vi "sectors checker.vi"(8 "error in (no error)":errorcluster, 10 "sections 2":string[][](array[string]), 11 "sections 1":string[][](array[string])) -> (0 "error out":errorcluster)   [LabVIEW 2024]
doc: "This VI compares the sections of two configuration files. The section names from each file are stored in the arrays <b>sections 1</b> and <b>sections 2</b>."
uses:
  443d4004-14de-444d-9e4b-623f00349db9.vi
  <vilib>/Utility/error.llb/Error Cluster From Error Code.vi
  <vilib>/ErrorRing/Error Ring.xnode
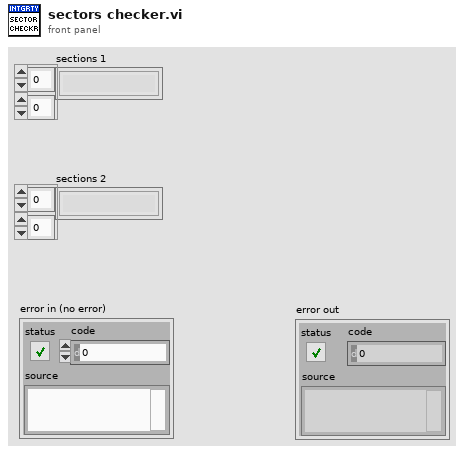
[diagram p1: front panel]
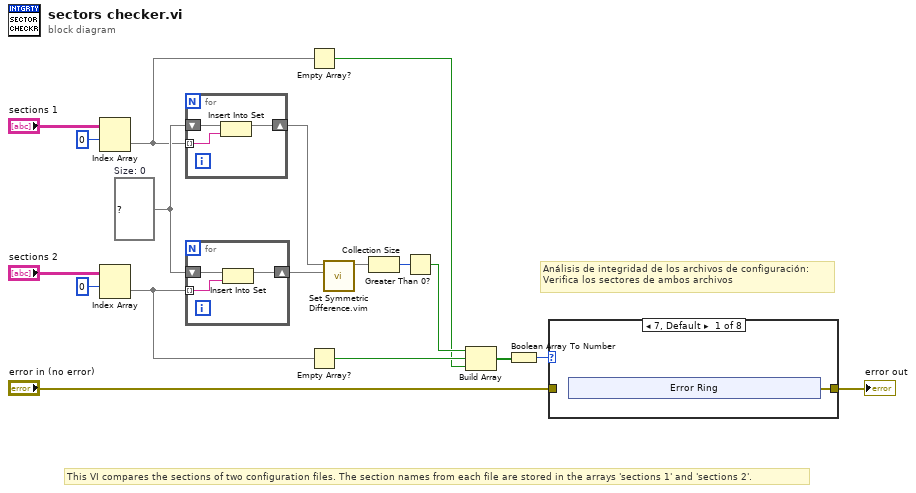
[diagram p0: block diagram]
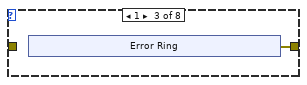
[diagram p3: hidden frame]
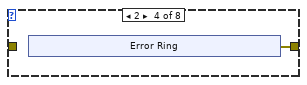
[diagram p4: hidden frame]
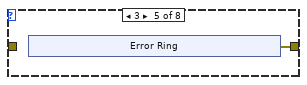
[diagram p5: hidden frame]
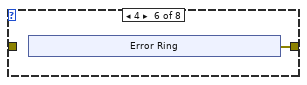
[diagram p6: hidden frame]
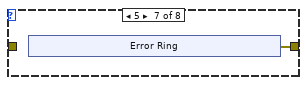
[diagram p7: hidden frame]
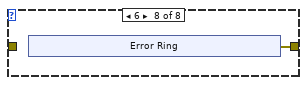
[diagram p8: hidden frame]
diagram:
  w15 = set{string} {}  # Size: 0
  # "This VI compares the sections of two configuration files. The section names from each file are stored in the arrays 'sections 1' and 'sections 2'."
  # "Análisis de integridad de los archivos de configuración:\nVerifica los sectores de ambos archivos"
  n1 = Index Array(array="sections 1", index (row)=0) -> (element=w1:string[])  [unwired: 1 in]
  n2 = Index Array(array="sections 2", index (row)=0) -> (element=w4:string[])  [unwired: 1 in]
  n3 = for {
    shift-right: [w20] -> w14
    shift-left: w15 -> [w21]
    tunnel: w1 -> [w19] mode=indexing
    n4 = Insert Into Set(10:w19, 11:w21) -> (3:w20:set{string})  [unwired: 1 out]
  }
  n5 = for {
    shift-right: [w23] -> w13
    shift-left: w15 -> [w24]
    tunnel: w4 -> [w22] mode=indexing
    n6 = Insert Into Set(10:w22, 11:w24) -> (3:w23:set{string})  [unwired: 1 out]
  }
  n7 = Empty Array?(array=w1) -> (empty?=w2:bool)
  n8 = Empty Array?(array=w4) -> (empty?=w3:bool)
  n9 = call "Set Symmetric Difference.vim"("set 2"=w13, "set 1"=w14) -> ("symmetric difference"=w12:set{string})  [unwired: 9 in]
  n10 = Collection Size(1:w12) -> (0:w11:i32)
  n11 = Greater Than 0?(x=w11) -> (x > 0?=w5:bool)
  n12 = Build Array(w5, w3, w2) -> (w9:bool[])
  n13 = Boolean Array To Number(Boolean array=w9) -> (number=w8:u32)
  n14 = case shown="7, Default" w8 {
    tunnel: "error in (no error)" -> [_ w31 _ _ _ _ _ _]
    tunnel: [w25 w31 w32 w38 w44 w50 w56 w62] -> w6
    frame 7, Default {
      n15 = xnode ("Error Ring")() -> ("error out"=w25:errorcluster)
    }
    frame 0 {
    }
    frame 1 {
      n16 = xnode ("Error Ring")() -> ("error out"=w32:errorcluster)
    }
    frame 2 {
      n17 = xnode ("Error Ring")() -> ("error out"=w38:errorcluster)
    }
    frame 3 {
      n18 = xnode ("Error Ring")() -> ("error out"=w44:errorcluster)
    }
    frame 4 {
      n19 = xnode ("Error Ring")() -> ("error out"=w50:errorcluster)
    }
    frame 5 {
      n20 = xnode ("Error Ring")() -> ("error out"=w56:errorcluster)
    }
    frame 6 {
      n21 = xnode ("Error Ring")() -> ("error out"=w62:errorcluster)
    }
  }
  "error out" <- w6
